vi "CreateClass.vi"(7 "PythonConverter_BD in":refnum<class "PyConvBD.lvclass">, 8 "error in":errorcluster, 11 "DiagramDisable in":refnum<class "DiagramDisable.lvclass">) -> (0 "error out":errorcluster, 3 "DiagramDisable out":refnum<class "DiagramDisable.lvclass">, 4 "class":string, 5 "PythonConverter_BD out":refnum<class "PyConvBD.lvclass">)   [LabVIEW 2014, in "DiagramDisable.lvclass"]
uses:
  DiagramDisable.lvclass
  Python/PythonConverter_BD/PyConvBD.lvclass
  Structure/Structure.lvclass/Structure.ctl
  Diagram/Diagram.lvclass
  Python/Parsing/Python Functions.lvlib
  Structure/Structure.lvclass
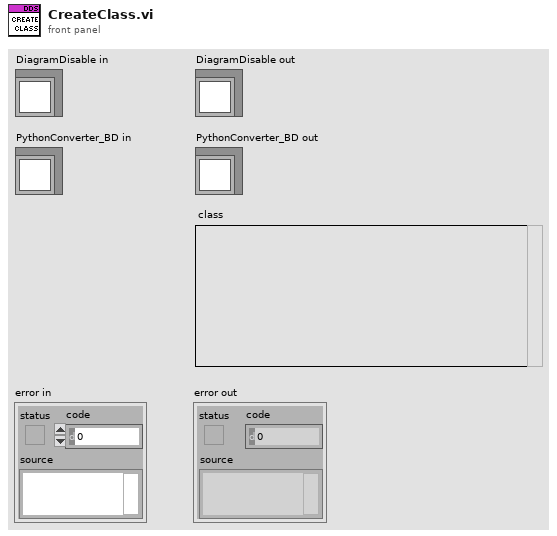
[diagram p1: front panel]
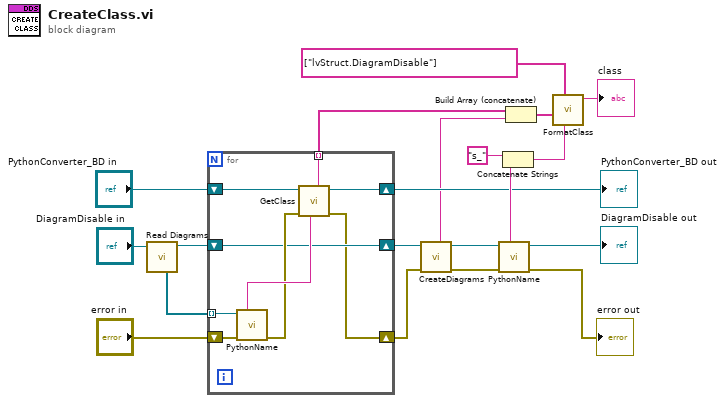
[diagram p0: block diagram]
diagram:
  n1 = call "Read Diagrams.vi"("Structure in"="DiagramDisable in") -> ("Structure out"=w13:refnum<class "DiagramDisable.lvclass">, "Diagrams"=w15:refnum<class "Diagram.lvclass">[])  [unwired: 7 in]
  n2 = for {
    tunnel: w15 -> [w29] mode=indexing
    shift-right: [w24] -> w12
    shift-left: "PythonConverter_BD in" -> [w28]
    shift-right: [w25] -> w11
    shift-left: w13 -> [w25]
    tunnel: [w23] -> w6 mode=indexing
    shift-right: [w21] -> w7
    shift-left: "error in" -> [w22]
    n3 = call-dynamic "PythonName.vi"("error in"=w22, "Diagram in"=w29) -> ("error out"=w26:errorcluster, "UID"=w27:string)  [unwired: 6 in, 2 out]
    n4 = call "GetClass.vi"("name"=w27, "error in"=w26, "PythonConverter_BD in"=w28) -> ("error out"=w21:errorcluster, "PythonConverter_BD out"=w24:refnum<class "PyConvBD.lvclass">, "class"=w23:string)  [unwired: 4 in]
  }
  "PythonConverter_BD out" <- w12
  n5 = call-dynamic "CreateDiagrams.vi"("error in"=w7, "Structure in"=w11) -> ("error out"=w1:errorcluster, "Structure out"=w2:refnum<class "DiagramDisable.lvclass">, "create_diagrams"=w5:string)  [unwired: 5 in]
  n6 = call-dynamic "PythonName.vi"("error in"=w1, "Node in"=w2) -> ("error out"=→"error out":errorcluster, "Node out"=→"DiagramDisable out":refnum<class "DiagramDisable.lvclass">, "UID"=w18:string)  [unwired: 6 in, 1 out]
  n7 = Concatenate Strings("s_" ("format string"), w18) -> (w17:string)
  n8 = Build Array (concatenate)(w6, w5) -> (w4:string[])
  n9 = call "FormatClass.vi"("name"=w17, "parameters/ancestors"=string[] ["lvStruct.DiagramDisable"], "body"=w4) -> ("python"=→"class":string)  [unwired: 8 in]
